vi "CreateWorkBook.vi"(8 "error":errorcluster caption="错误输入（无错误）", 10 "FileName":string, 11 "Excel.Workbooks":refnum<k7>) -> (0 "错误输出":errorcluster, 3 "Excel.Workbooks":refnum<k7>)   [LabVIEW 2014]
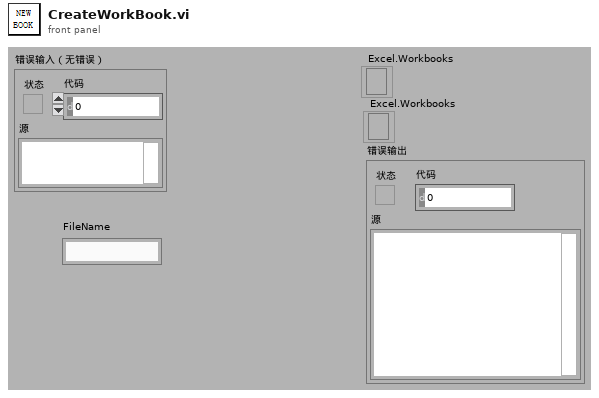
[diagram p1: front panel]
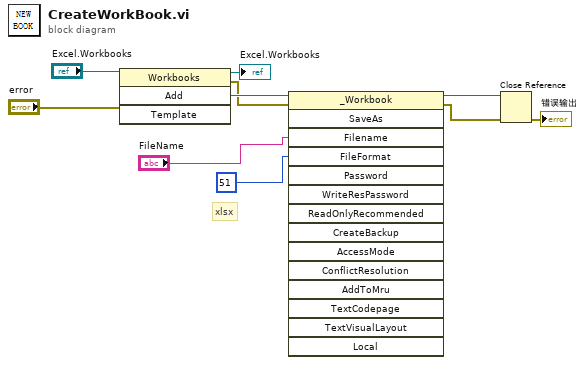
[diagram p0: block diagram]
diagram:
  # "xlsx"
  n1 = invoke class="Workbooks" method="Add"(reference="Excel.Workbooks", error in="error") -> (reference out=→"Excel.Workbooks":refnum<k7>, error out=w4:errorcluster, "Add"=w9:refnum<k7>)  [unwired: 2 in, 1 out]
  n2 = invoke class="_Workbook" method="SaveAs"(reference=w9, error in=w4, "Filename"="FileName", "FileFormat"=51) -> (reference out=w6:refnum<k7>, error out=w5:errorcluster)  [unwired: 11 in, 13 out]
  n3 = Close Reference(reference=w6, error in (no error)=w5) -> (error out=→"错误输出":errorcluster)
